vi "Teleop.vi"(10 "Match Info":T1={"Autonomous Elapsed Seconds"=0.0, "TeleOp Elapsed Seconds"=0.0, "Disabled Elapsed Seconds"=0.0, "Visited Autonomous"=FALSE, "Visited TeleOp"=FALSE, "Visited Disabled"=FALSE, "Autonomous Settings"={"Autonomous Style"=enum."Independent", "VI Refnum"=refnum}}, 11 "Call Context":T2) -> ()   [LabVIEW 2015]
doc: "This VI is called for each TeleOp packet received from the DS where the robot is not disabled. It is often used to read from the joysticks and update I/O or to update setpoints for timed control loops. It should complete and return within 20 milliseconds or it may miss DS packets."
uses:
  <vilib>/Rock Robotics/WPI/DriverStation/WPI_DriverStationDerivedRobotMode.ctl
  <vilib>/Rock Robotics/WPI/DriverStation/WPI_DriverStationMatch Info.ctl
  <vilib>/Rock Robotics/WPI/Solenoid/WPI_SolenoidValue.ctl
  <vilib>/Rock Robotics/Network Tables/NT Write Boolean.vi
  <vilib>/Rock Robotics/WPI/Solenoid/WPI_SolenoidSetEnum.vi
  Robot Global Data.vi
  hhVI/hhVI.lvlib
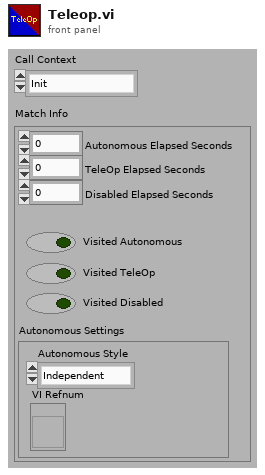
[diagram p1: front panel]
types:
  T1 = typedef "WPI_DriverStationMatch Info.ctl" = cluster{"Autonomous Elapsed Seconds":dbl, "TeleOp Elapsed Seconds":dbl, "Disabled Elapsed Seconds":dbl, "Visited Autonomous":bool, "Visited TeleOp":bool, "Visited Disabled":bool, "Autonomous Settings":cluster{"Autonomous Style":enum16{"Iterative", "Independent"}, "VI Refnum":refnum<vi>}}
  T2 = typedef "WPI_DriverStationDerivedRobotMode.ctl" = enum16{"Init", "Execute", "Stop"}
  T3 = typedef "WPI_SolenoidValue.ctl" = enum16{"Off", "On", "Forward", "Reverse"}
  T4 = typedef "WPI_SolenoidDevRef.ctl" = cluster{"DevStatus":errorcluster, "Pneumatics Control Module":u8, "Forward Solenoid Channel":T5, "Reverse Solenoid Channel":T5}
  T5 = typedef "WPI_SolenoidChannel.ctl" = enum8{"Solenoid 0", "Solenoid 1", "Solenoid 2", "Solenoid 3", "Solenoid 4", "Solenoid 5", "Solenoid 6", "Solenoid 7", "Invalid"}
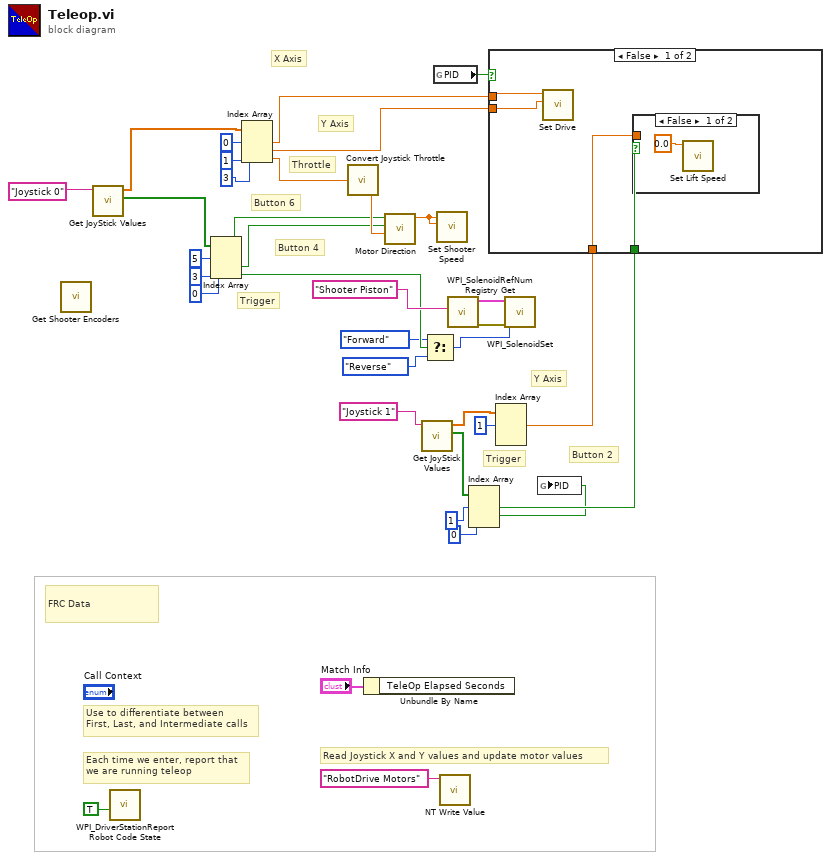
[diagram p0: block diagram]
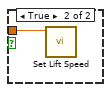
[diagram p2: hidden frame]
diagram:
  # "Trigger"
  # "FRC Data"
  # "Button 2"
  # "Trigger"
  # "Y Axis"
  # "Button 4"
  # "Button 6"
  # "Throttle"
  # "Y Axis"
  # "X Axis"
  # "Each time we enter, report that\nwe are running teleop"
  # "Use to differentiate between\nFirst, Last, and Intermediate calls"
  # "Read Joystick X and Y values and update motor values"
  n1 = call "Get Shooter Encoders.vi"() -> ()  [unwired: 10 in, 2 out]
  n2 = call "Get JoyStick Values.vi"("Joystick Name"="Joystick 0" ("refnum name")) -> ("Buttons"=w20:bool[], "Axes"=w25:dbl[])  [unwired: 9 in]
  n3 = call <vilib>:"WPI_DriverStationReport Robot Code State.vi"("TeleOp"=TRUE ("Autonomous")) -> ()  [unwired: 10 in, 1 out]
  n4 = Index Array(array=w20, index #1=5 ("index"), index #2=3 ("index"), index #3=0 ("index")) -> (element #1=w21:bool, element #2=w18:bool, element #3=w7:bool)
  n5 = Index Array(array=w25, index #1=0 ("index"), index #2=1 ("index"), index #3=3 ("index")) -> (element #1=w27:dbl, element #2=w28:dbl, element #3=w19:dbl)
  n6 = call "Convert Joystick Throttle.vi"("Input"=w19) -> ("Output"=w32:dbl)
  n7 = Unbundle By Name("Match Info") -> ()  [unwired: 1 out]
  n8 = call "Motor Direction.vi"("Speed"=w32, "Backwards"=w18, "Forward"=w21) -> ("Direction"=w31:dbl)  [unwired: 8 in]
  n9 = call "Get JoyStick Values.vi"("Joystick Name"="Joystick 1" ("refnum name")) -> ("Buttons"=w12:bool[], "Axes"=w17:dbl[])  [unwired: 9 in]
  n10 = Select(t=WPI_SolenoidValue."Forward" ("Value"), s=w7, f=WPI_SolenoidValue."Reverse" ("Value")) -> (s? t:f=w6:T3)
  n11 = global read "Robot Global Data.vi" "PID"() -> (w33:bool)
  n12 = call "Set Shooter Speed.vi"("Set Bottom Speed"=w31, "Set Top Speed"=w31) -> ()  [unwired: 10 in]
  n13 = call-poly <vilib>:"NT Write Value.vi"("Name"="RobotDrive Motors") -> ()  [unwired: 10 in, 1 out]
  n14 = call <vilib>:"WPI_SolenoidRefNum Registry Get.vi"("refnum name"="Shooter Piston") -> ("error out"=w10:errorcluster, "SolenoidDevRef"=w9:T4)  [unwired: 9 in]
  n15 = Index Array(array=w12, index #1=1 ("index"), index #2=0 ("index")) -> (element #1=w13:bool, element #2=w1:bool)  [unwired: 1 in, 1 out]
  n16 = Index Array(array=w17, index #1=1 ("index")) -> (element #1=w15:dbl)  [unwired: 2 in, 2 out]
  n17 = case shown="False" w33 {
    tunnel: w28 -> [w38 _]
    tunnel: w27 -> [w37 _]
    tunnel: w15 -> [w40 _]
    tunnel: w13 -> [w39 _]
    frame False {
      n18 = call "Set Drive.vi"("Y axis value"=w38, "X axis value"=w37) -> ()  [unwired: 10 in]
      n19 = case shown="False" w39 {
        tunnel: w40 -> [_ w42]
        frame False {
          n20 = call "Set Lift Speed.vi"("Speed"=0.0) -> ()  [unwired: 11 in]
        }
        frame True {
          n21 = call "Set Lift Speed.vi"("Speed"=w42) -> ()  [unwired: 11 in]
        }
      }
    }
    frame True {
    }
  }
  n22 = call-poly <vilib>:"WPI_SolenoidSet.vi"("error in (no error)"=w10, "Value"=w6, "SolenoidDevRef"=w9) -> ()  [unwired: 7 in, 2 out]
  n23 = global write "Robot Global Data.vi" "PID"(w1) -> ()
